vi "RetroParseGate.vi"(11 "Choose Directory":path) -> ()   [LabVIEW 2022 SP3]
panel:
  out "Raw data":i16[][](graph)
  out "Root Name":string
  out "File num":i32
  in  "Use Selected Files":bool
  in  "Listbox":i32[](listbox)
  in  "file ext":string="000"
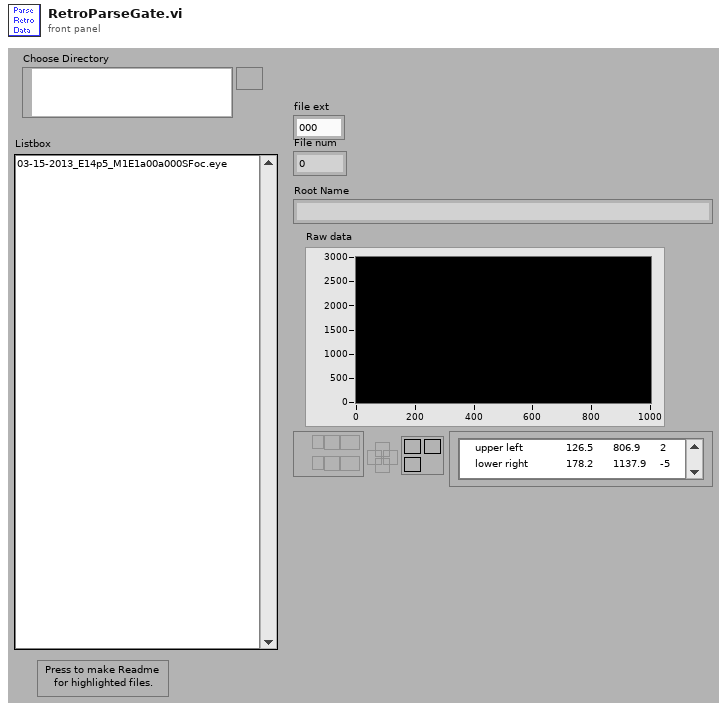
[diagram p1: front panel]
types:
  T1 = enum16{"open", "replace", "create", "open or create", "replace or create", "replace or create with confirmation"}
  T2 = enum16{"big-endian, network order", "native, host order", "little-endian"}
  T3 = cluster{"# rf points per line":u16, "# lines per scan":u16, "sample rate MHz":u16, "# A/D bits":i16, "# bytes per A/D":u16, "TGC Flag":u16, "A/D Type":string}
  T4 = typedef "Header.ctl" = cluster{"header info":cluster{"Header":string, "Head length":i16}, "A/D info":cluster{"# rf points per line":u16, "# lines per scan":u16, "sample rate MHz":u16, "# A/D bits":i16, "# bytes per A/D":u16, "TGC Flag":u16, "A/D Type":string}, "Tranducer Info":cluster{"bandwidth":sgl, "center freq":sgl, "start freq":sgl, "ID":i32}, "Scan Info":cluster{"delay":sgl, "pivot distance":sgl, "sector scan angle":sgl, "operator":string, "Scan Mode":string, "location":string}, "Time/Date Info":cluster{"date":string, "time":string}, "RF Info":cluster{"RF file name":string, "RF file att":string, "RF cal file name":string, "RF cal file att":string}, "Patient Info":cluster{"ID":string, "extended ID":string, "age":u16, "sex":string, "previously\nscanned":string, "PSA":sgl, "LOS":u8, "Ethnicty 2":u8, "Race":u8}, "Tissue Type":cluster{"organ":i16, "disease type":i16, "disease location":i16, "IQ_pts":u16, "RcvBuffer":u8, "RcvFrame":u16, "IQBuff":u8, "IQFrame":u16, "IQPage":u8}, "Votage scaling":cluster{"Digitizer (dB)":sgl, "Gain (dB)":sgl, "Atten (dB)":sgl}, "Comment":string, "Misc Info":cluster{"avg num":u16, "c speed":i16, "Div By or SF zones":i16, "XMIT CHS":u8, "RCV CHS":u8, "Xmit angle":sgl}, "Therapy Parameters":cluster{"Theraputic Freq (MHz)":sgl, "Time on (s)":sgl, "Therapy amplitude (mV)":sgl, "Lines Before":u16, "Lines After":u16}, "Scan Settings":cluster{"Energy (uJ or V)":u8, "Damp (Ohm) or Fc":u8, "HP Filt (KHz)":u8, "LP Filt (MHz)":u8, "Gain (db)":u8, "prf (kHz)":sgl, "Distance between\nscan lines (um)":u16, "Distance between\nscan planes (um)":u16, "Scan line gap (um)":sgl, "Scan plane gap (um)":sgl}, "Compression Parameters":cluster{"F1 (MHz)":sgl, "F2 (MHz)":sgl, "% taper":sgl, "duration":sgl}, "Patient Info Xtra":cluster{"First Name":string, "Last Name":string, "Notes":string}, "ROI Box":u16[]}
  T5 = cluster{"Energy (microJ)":u8, "Damping (In Ohm)":u8, "HP Filt(KHz) ":u8, "LP Filt (MHz)":u8, "Gain (db)":u8, "prf (kHz)":sgl, "Distance between\nscan lines (mm)":u16, "Distance between\nscan planes (mm)":u16}
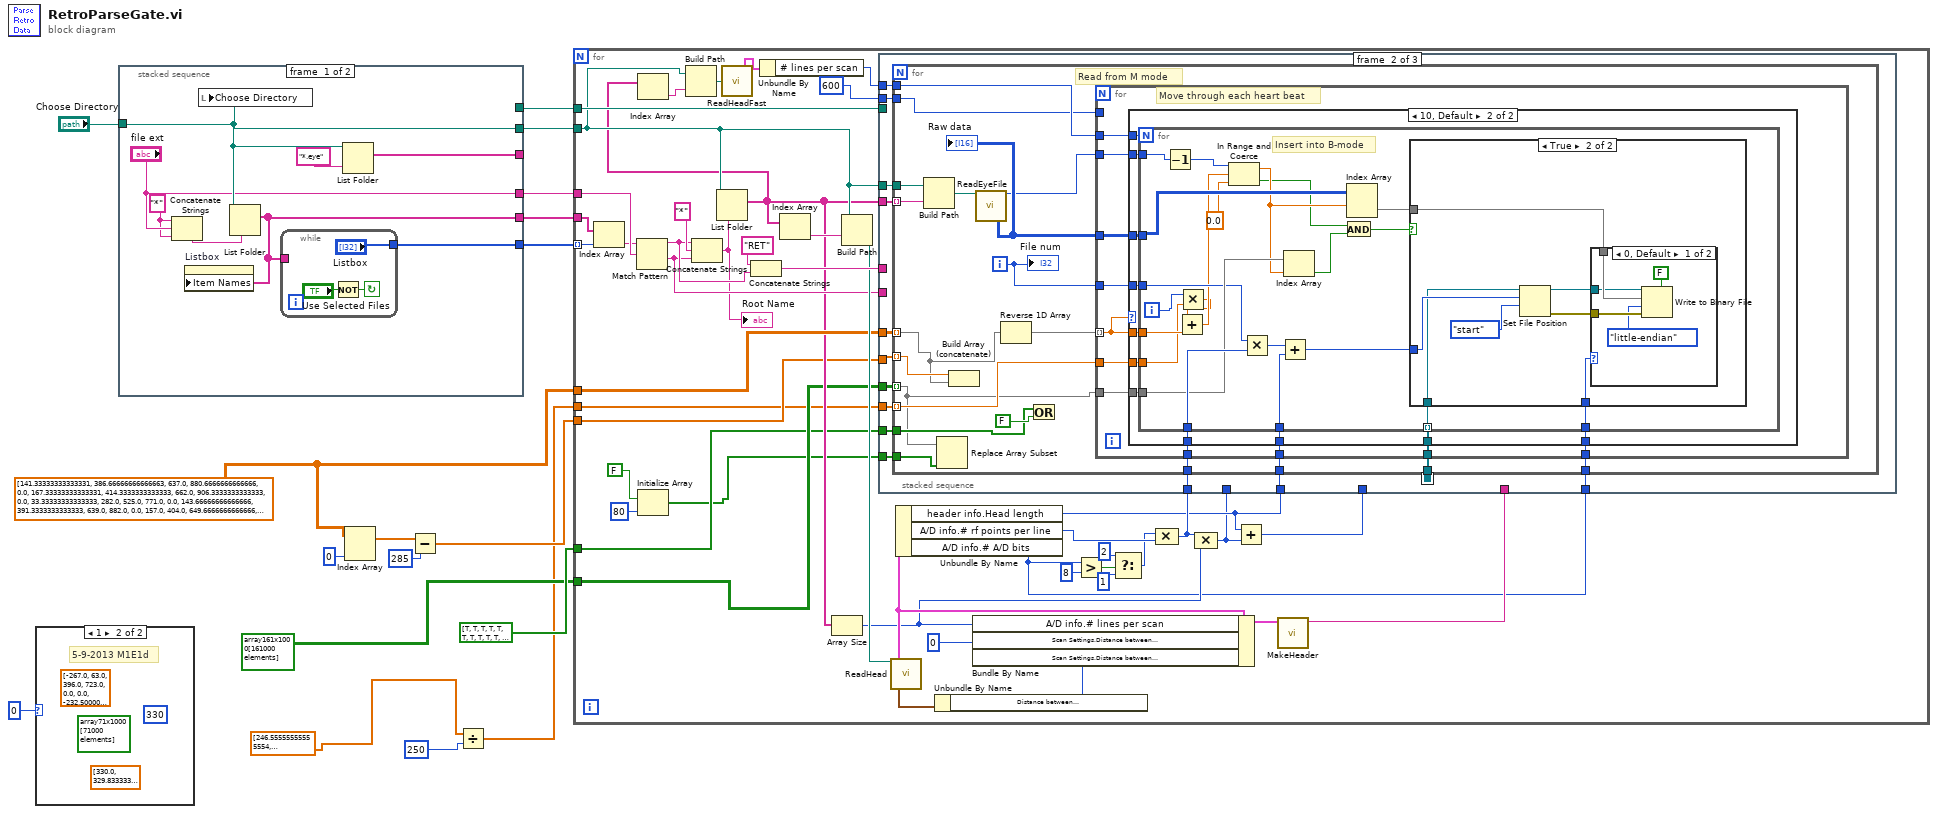
[diagram p0: block diagram]
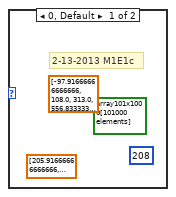
[diagram p2: hidden frame]
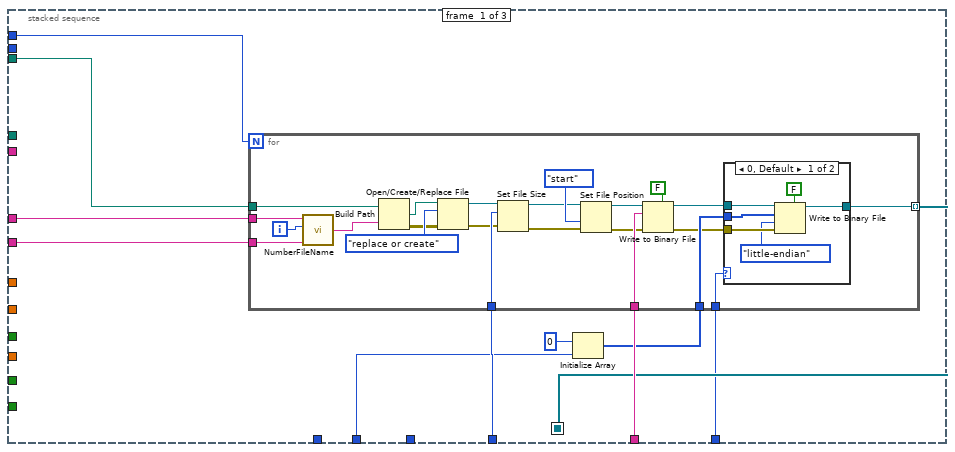
[diagram p3: hidden frame]
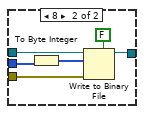
[diagram p4: hidden frame]
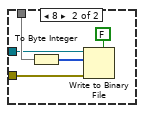
[diagram p7: hidden frame]
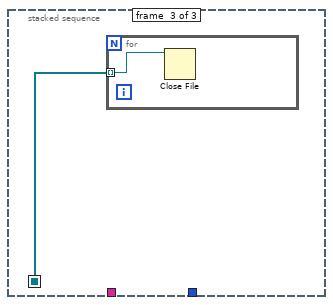
[diagram p8: hidden frame]
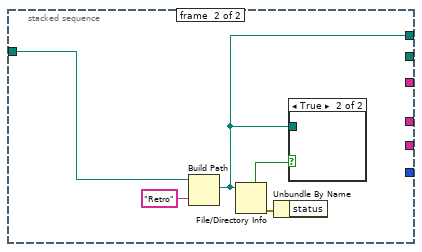
[diagram p9: hidden frame]
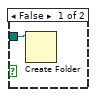
[diagram p10: hidden frame]
diagram:
  w3 = dbl[][] [[141.33333333333331, 386.66666666666663, 637.0, 880.6666666666666, 0.0], [167.33333333333331, 414.3333333333333, 662.0, 906.3333333333333, 0.0], [33.33333333333333, 282.0, 525.0, 771.0, 0.0], [143.66666666666666, 391.3333333333333, 639.0, 882.0, 0.0], [157.0, 404.0, 649.6666666666666, 893.6666666666666, 0.0], [157.66666666666666, 403.66666666666663, 651.0, 893.0, 0.0], [34.33333333333333, 283.66666666666663, 523.6666666666666, 767.6666666666666, 0.0], [120.0, 363.3333333333333, 607.6666666666666, 851.0, 0.0], [119.66666666666666, 364.0, 607.0, 853.0, 0.0], [117.0, 359.0, 604.3333333333333, 845.6666666666666, 0.0], [103.0, 347.3333333333333, 589.0, 833.6666666666666, 0.0], [124.0, 368.3333333333333, 612.6666666666666, 853.6666666666666, 0.0], [134.33333333333331, 376.0, 618.3333333333333, 860.6666666666666, 0.0], [120.0, 360.66666666666663, 604.3333333333333, 846.3333333333333, 0.0], [85.66666666666666, 328.66666666666663, 570.3333333333333, 816.3333333333333, 0.0], [96.66666666666666, 337.66666666666663, 579.6666666666666, 824.0, 0.0], [65.66666666666666, 306.66666666666663, 547.6666666666666, 789.6666666666666, 0.0], [26.333333333333332, 270.66666666666663, 512.3333333333333, 753.3333333333333, 0.0], [127.0, 369.0, 610.6666666666666, 854.6666666666666, 0.0], [142.33333333333331, 385.3333333333333, 627.0, 868.0, 0.0], [177.33333333333331, 420.0, 660.0, 901.6666666666666, 0.0], [192.33333333333331, 436.66666666666663, 678.3333333333333, 921.0, 0.0], [215.33333333333331, 458.3333333333333, 701.6666666666666, 944.3333333333333, 0.0], [20.333333333333332, 266.66666666666663, 508.66666666666663, 752.0, 0.0], [55.666666666666664, 300.3333333333333, 543.6666666666666, 787.3333333333333, 0.0], [73.33333333333333, 317.0, 560.0, 804.0, 0.0], [91.66666666666666, 336.3333333333333, 578.6666666666666, 820.6666666666666, 0.0], [120.33333333333333, 362.66666666666663, 606.0, 847.0, 0.0], [177.33333333333331, 419.0, 660.6666666666666, 902.0, 0.0], [191.66666666666666, 435.0, 673.3333333333333, 916.0, 0.0], [204.33333333333331, 445.0, 925.0, 0.0, 0.0], [235.0, 472.0, 712.0, 951.6666666666666, 0.0], [45.0, 282.66666666666663, 522.6666666666666, 760.3333333333333, 0.0], [66.66666666666666, 305.3333333333333, 547.0, 784.6666666666666, 0.0], [45.0, 282.0, 522.0, 763.3333333333333, 0.0], [77.0, 315.66666666666663, 556.0, 794.6666666666666, 0.0], [110.66666666666666, 349.3333333333333, 586.0, 827.0, 0.0], [135.33333333333331, 376.0, 612.3333333333333, 852.0, 0.0], [159.66666666666666, 400.3333333333333, 635.3333333333333, 877.6666666666666, 0.0], [141.0, 378.0, 615.6666666666666, 856.6666666666666, 0.0], [127.66666666666666, 366.0, 603.3333333333333, 843.3333333333333, 0.0], [149.66666666666666, 386.66666666666663, 622.6666666666666, 863.6666666666666, 0.0], [92.33333333333333, 328.0, 567.3333333333333, 808.3333333333333, 0.0], [79.66666666666666, 316.3333333333333, 553.6666666666666, 792.6666666666666, 0.0], [30.0, 266.3333333333333, 505.66666666666663, 742.0, 0.0], [9.333333333333332, 247.0, 486.66666666666663, 726.3333333333333, 960.0], [15.666666666666666, 252.33333333333331, 492.3333333333333, 727.6666666666666, 0.0], [197.0, 437.0, 672.0, 910.6666666666666, 0.0], [171.66666666666666, 411.3333333333333, 648.3333333333333, 887.3333333333333, 0.0], [149.0, 385.0, 623.3333333333333, 861.0, 0.0], [126.33333333333333, 363.3333333333333, 597.6666666666666, 837.0, 0.0], [111.0, 348.0, 581.6666666666666, 820.3333333333333, 0.0], [89.66666666666666, 321.66666666666663, 559.0, 799.0, 0.0], [77.33333333333333, 312.3333333333333, 548.6666666666666, 786.3333333333333, 0.0], [28.333333333333332, 262.3333333333333, 503.0, 737.0, 0.0], [92.66666666666666, 328.66666666666663, 567.0, 802.6666666666666, 0.0], [32.666666666666664, 267.0, 506.0, 740.3333333333333, 0.0], [188.0, 424.0, 658.3333333333333, 897.6666666666666, 0.0], [151.33333333333331, 386.66666666666663, 620.6666666666666, 860.6666666666666, 0.0], [341.3333333333333, 576.0, 0.0, 0.0, 0.0], [52.33333333333333, 285.3333333333333, 529.3333333333333, 759.6666666666666, 0.0], [238.33333333333331, 714.0, 949.0, 0.0, 0.0], [49.33333333333333, 285.0, 518.3333333333333, 757.6666666666666, 0.0], [80.33333333333333, 314.0, 552.0, 789.0, 0.0], [70.0, 305.0, 593.0, 777.0, 0.0], [228.66666666666666, 464.3333333333333, 701.3333333333333, 937.0, 0.0], [183.0, 654.3333333333333, 890.6666666666666, 0.0, 0.0], [134.66666666666666, 369.3333333333333, 603.0, 0.0, 0.0], [46.0, 282.0, 517.0, 752.0, 0.0], [231.66666666666666, 469.3333333333333, 702.0, 938.0, 0.0], [213.0, 679.6666666666666, 919.6666666666666, 0.0, 0.0], [27.666666666666664, 262.3333333333333, 498.0, 733.3333333333333, 966.3333333333333], [186.0, 421.66666666666663, 654.0, 892.6666666666666, 0.0], [143.0, 376.66666666666663, 611.3333333333333, 0.0, 0.0], [193.66666666666666, 662.3333333333333, 898.6666666666666, 0.0, 0.0], [120.0, 354.0, 589.0, 0.0, 0.0], [156.0, 623.0, 0.0, 0.0, 0.0], [314.66666666666663, 555.0, 0.0, 0.0, 0.0], [110.0, 344.0, 578.0, 815.0, 0.0], [134.0, 602.3333333333333, 0.0, 0.0, 0.0], [170.33333333333331, 638.0, 0.0, 0.0, 0.0], [131.33333333333331, 366.0, 600.6666666666666, 833.3333333333333, 0.0], [5.333333333333333, 237.33333333333331, 472.66666666666663, 709.3333333333333, 939.3333333333333], [164.66666666666666, 401.66666666666663, 634.6666666666666, 866.0, 0.0], [165.66666666666666, 399.0, 633.0, 866.0, 0.0], [150.33333333333331, 384.0, 620.3333333333333, 853.6666666666666, 0.0], [102.33333333333333, 336.0, 570.6666666666666, 804.6666666666666, 0.0], [65.66666666666666, 300.0, 532.6666666666666, 767.3333333333333, 0.0], [52.0, 288.3333333333333, 519.6666666666666, 752.6666666666666, 0.0], [56.0, 293.3333333333333, 525.0, 756.6666666666666, 0.0], [225.33333333333331, 458.3333333333333, 703.3333333333333, 926.0, 0.0], [170.33333333333331, 402.66666666666663, 636.6666666666666, 873.3333333333333, 0.0], [115.66666666666666, 347.3333333333333, 582.6666666666666, 815.6666666666666, 0.0], [27.666666666666664, 261.66666666666663, 496.0, 729.3333333333333, 962.3333333333333], [188.66666666666666, 420.3333333333333, 655.3333333333333, 889.0, 0.0], [152.0, 385.66666666666663, 618.3333333333333, 853.6666666666666, 0.0], [159.66666666666666, 391.0, 626.0, 858.6666666666666, 0.0], [158.0, 392.66666666666663, 624.3333333333333, 858.3333333333333, 0.0], [103.33333333333333, 336.66666666666663, 570.6666666666666, 803.0, 0.0], [39.666666666666664, 275.66666666666663, 506.66666666666663, 751.6666666666666, 0.0], [194.0, 426.3333333333333, 659.6666666666666, 893.6666666666666, 0.0], [139.33333333333331, 371.3333333333333, 604.0, 837.3333333333333, 0.0], [85.66666666666666, 319.3333333333333, 553.3333333333333, 784.6666666666666, 0.0], [220.0, 453.0, 687.3333333333333, 920.6666666666666, 0.0], [118.66666666666666, 352.66666666666663, 586.6666666666666, 819.3333333333333, 0.0], [40.0, 274.66666666666663, 506.66666666666663, 738.3333333333333, 0.0], [16.333333333333332, 249.0, 485.0, 716.3333333333333, 950.3333333333333], [200.33333333333331, 434.0, 668.0, 900.3333333333333, 0.0], [102.0, 333.66666666666663, 566.0, 797.6666666666666, 0.0], [32.33333333333333, 267.3333333333333, 499.0, 734.6666666666666, 964.0], [208.33333333333331, 443.3333333333333, 675.3333333333333, 908.3333333333333, 0.0], [94.0, 326.3333333333333, 560.3333333333333, 794.6666666666666, 0.0], [205.0, 438.0, 671.3333333333333, 904.6666666666666, 0.0], [90.66666666666666, 328.3333333333333, 557.6666666666666, 790.6666666666666, 0.0], [206.66666666666666, 439.3333333333333, 672.6666666666666, 907.3333333333333, 0.0], [149.0, 383.3333333333333, 613.0, 849.6666666666666, 0.0], [74.66666666666666, 303.66666666666663, 540.0, 775.6666666666666, 0.0], [193.33333333333331, 427.3333333333333, 659.3333333333333, 893.3333333333333, 0.0], [75.33333333333333, 307.66666666666663, 541.3333333333333, 772.6666666666666, 0.0], [227.66666666666666, 459.3333333333333, 927.0, 0.0, 0.0], [171.0, 404.66666666666663, 637.0, 869.6666666666666, 0.0], [67.0, 533.3333333333333, 766.3333333333333, 0.0, 0.0], [145.33333333333331, 376.66666666666663, 611.3333333333333, 846.3333333333333, 0.0], [220.0, 452.0, 685.0, 917.3333333333333, 0.0], [140.66666666666666, 373.0, 605.6666666666666, 839.6666666666666, 0.0], [47.33333333333333, 291.0, 515.3333333333333, 750.3333333333333, 0.0], [184.33333333333331, 419.0, 651.3333333333333, 886.0, 0.0], [102.0, 335.0, 567.0, 800.6666666666666, 0.0], [166.0, 399.3333333333333, 630.3333333333333, 864.0, 0.0], [10.0, 243.33333333333331, 476.66666666666663, 709.0, 943.6666666666666], [103.33333333333333, 335.66666666666663, 570.3333333333333, 802.6666666666666, 0.0], [12.0, 245.0, 477.3333333333333, 711.6666666666666, 946.0], [79.0, 318.66666666666663, 547.3333333333333, 780.0, 0.0], [158.33333333333331, 392.0, 626.3333333333333, 859.6666666666666, 0.0], [21.0, 254.33333333333331, 490.0, 721.6666666666666, 954.6666666666666], [139.33333333333331, 369.66666666666663, 604.0, 836.6666666666666, 0.0], [223.33333333333331, 458.3333333333333, 691.6666666666666, 924.3333333333333, 0.0], [38.0, 272.66666666666663, 504.3333333333333, 741.6666666666666, 0.0], [54.33333333333333, 522.0, 759.6666666666666, 0.0, 0.0], [144.33333333333331, 376.3333333333333, 611.3333333333333, 846.6666666666666, 0.0], [12.0, 244.33333333333331, 478.66666666666663, 711.3333333333333, 945.6666666666666], [78.0, 544.0, 778.3333333333333, 0.0, 0.0], [131.33333333333331, 363.3333333333333, 597.0, 830.0, 0.0], [141.0, 373.0, 606.6666666666666, 842.0, 0.0], [188.33333333333331, 422.3333333333333, 654.3333333333333, 887.3333333333333, 0.0], [53.666666666666664, 521.0, 758.0, 0.0, 0.0], [134.33333333333331, 365.3333333333333, 600.0, 832.6666666666666, 0.0], [218.33333333333331, 451.66666666666663, 686.6666666666666, 920.0, 0.0], [8.666666666666666, 240.0, 473.3333333333333, 708.3333333333333, 940.3333333333333], [217.66666666666666, 451.66666666666663, 686.6666666666666, 917.3333333333333, 0.0], [238.66666666666666, 470.0, 705.6666666666666, 940.0, 0.0], [50.33333333333333, 287.3333333333333, 519.3333333333333, 762.6666666666666, 0.0], [109.0, 343.66666666666663, 574.6666666666666, 810.0, 0.0], [160.0, 392.66666666666663, 626.6666666666666, 859.3333333333333, 0.0], [170.66666666666666, 403.3333333333333, 639.0, 869.0, 0.0], [139.33333333333331, 371.0, 836.0, 0.0, 0.0], [152.33333333333331, 383.3333333333333, 621.6666666666666, 851.6666666666666, 0.0], [236.33333333333331, 471.66666666666663, 700.6666666666666, 935.6666666666666, 0.0], [23.666666666666664, 258.0, 491.66666666666663, 725.6666666666666, 957.0], [226.33333333333331, 459.66666666666663, 693.3333333333333, 924.6666666666666, 0.0], [212.33333333333331, 443.0, 677.0, 911.0, 0.0]] ("Beat INput")
  n1 = case shown="1" 0 {
    frame 0, Default {
      (unwired) 208
      (unwired) dbl[] [205.91666666666666, 210.27777777777777, 205.88888888888889, 208.66666666666666, 207.25, 211.72222222222223, 206.77777777777774, 211.54166666666666, 208.83333333333331, 212.27777777777774, 215.55555555555554, 212.25, 215.7222222222222, 217.04166666666666, 213.38888888888889, 217.875, 218.16666666666666, 163.375, 220.87499999999997, 219.77777777777777, 221.94444444444446, 221.5, 221.5, 224.27777777777777, 224.27777777777777, 224.5, 224.94444444444443, 222.54166666666666, 223.27777777777774, 223.625, 227.88888888888886, 223.88888888888886, 222.77777777777777, 222.83333333333331, 222.20833333333331, 223.16666666666666, 222.91666666666666, 223.11111111111111, 221.91666666666669, 223.33333333333331, 221.05555555555554, 221.7222222222222, 220.16666666666666, 221.70833333333331, 222.72222222222223, 220.77777777777774, 222.11111111111111, 220.66666666666666, 223.04166666666666, 223.27777777777777, 223.2222222222222, 223.66666666666666, 222.61111111111111, 227.27777777777774, 223.95833333333331, 225.88888888888886, 223.875, 226.45833333333334, 227.7222222222222, 224.88888888888889, 224.83333333333334, 223.375, 224.75, 223.0, 223.94444444444446, 223.54166666666666, 223.61111111111111, 225.94444444444443, 226.0, 225.87499999999997, 228.66666666666666, 230.72222222222223, 230.33333333333334, 226.20833333333334, 232.0, 231.55555555555554, 230.70833333333334, 232.66666666666666, 231.94444444444443, 230.2222222222222, 228.83333333333331, 229.79166666666666, 234.27777777777777, 233.16666666666666, 232.77777777777774, 229.16666666666666, 228.6111111111111, 234.55555555555557, 232.20833333333331, 232.05555555555557, 229.61111111111111, 231.6111111111111, 230.29166666666666, 230.29166666666669, 228.61111111111111, 231.1111111111111, 231.91666666666666, 232.49999999999997, 232.27777777777777, 231.27777777777774, 230.55555555555557] ("Array")
      (unwired) bool[][] array101x1000[101000 elements] ("Resp Gate")
      (unwired) dbl[][] [[-97.91666666666666, 108.0, 313.0, 556.8333333333333, 720.3333333333333, 931.6666666666666, 0.0], [-29.611111111111114, 180.66666666666666, 392.3333333333333, 603.5, 811.5, 0.0, 0.0], [-44.888888888888886, 161.0, 365.8333333333333, 624.1666666666666, 778.6666666666666, 0.0, 0.0], [-50.0, 158.66666666666666, 368.8333333333333, 573.1666666666666, 784.6666666666666, 0.0, 0.0], [-131.91666666666669, 75.33333333333333, 285.16666666666663, 492.66666666666663, 699.5, 904.3333333333333, 0.0], [-40.388888888888914, 171.33333333333331, 383.3333333333333, 596.0, 806.5, 0.0, 0.0], [-14.777777777777743, 192.0, 403.3333333333333, 636.8333333333333, 812.3333333333333, 0.0, 0.0], [-102.04166666666666, 109.5, 323.66666666666663, 545.1666666666666, 745.8333333333333, 955.6666666666666, 0.0], [-136.5, 72.33333333333333, 283.0, 493.0, 695.1666666666666, 907.6666666666666, 0.0], [-1.277777777777743, 211.0, 423.66666666666663, 635.1666666666666, 847.8333333333333, 0.0, 0.0], [3.444444444444457, 219.0, 434.3333333333333, 650.3333333333333, 865.6666666666666, 0.0, 0.0], [-89.41666666666667, 122.83333333333333, 330.3333333333333, 543.0, 758.6666666666666, 971.8333333333333, 0.0], [-73.2222222222222, 142.5, 358.5, 576.1666666666666, 789.6666666666666, 0.0, 0.0], [-196.70833333333331, 20.333333333333332, 238.16666666666666, 452.66666666666663, 671.3333333333333, 888.5, 0.0], [-9.888888888888886, 203.5, 440.8333333333333, 628.0, 843.6666666666666, 0.0, 0.0], [-117.875, 100.0, 318.5, 535.1666666666666, 752.0, 971.5, 0.0], [-141.66666666666666, 76.5, 316.3333333333333, 512.1666666666666, 730.3333333333333, 949.1666666666666, 0.0], [-37.54166666666667, 125.83333333333333, 345.0, 387.8333333333333, 559.1666666666666, 779.3333333333333, 0.0], [-197.54166666666663, 23.333333333333332, 245.66666666666666, 491.0, 686.3333333333333, 906.8333333333333, 0.0], [-24.444444444444457, 195.33333333333331, 416.0, 633.6666666666666, 854.6666666666666, 0.0, 0.0], [-185.2777777777778, 36.666666666666664, 258.66666666666663, 480.66666666666663, 702.5, 0.0, 0.0], [4.666666666666657, 226.16666666666666, 446.16666666666663, 669.6666666666666, 890.6666666666666, 0.0, 0.0], [-114.83333333333334, 106.66666666666666, 328.0, 547.6666666666666, 771.1666666666666, 0.0, 0.0], [-30.111111111111114, 194.16666666666666, 455.8333333333333, 643.3333333333333, 867.0, 0.0, 0.0], [-79.61111111111111, 144.66666666666666, 371.5, 595.8333333333333, 817.5, 0.0, 0.0], [-150.16666666666669, 74.33333333333333, 299.3333333333333, 524.3333333333333, 747.0, 972.3333333333333, 0.0], [-125.1111111111111, 99.83333333333333, 323.66666666666663, 547.8333333333333, 774.6666666666666, 0.0, 0.0], [-160.875, 61.666666666666664, 283.3333333333333, 507.5, 730.0, 951.8333333333333, 0.0], [-59.77777777777774, 163.5, 387.8333333333333, 610.3333333333333, 833.3333333333333, 0.0, 0.0], [-151.625, 72.0, 296.0, 549.0, 743.8333333333333, 966.5, 0.0], [-70.7222222222222, 157.16666666666666, 380.3333333333333, 603.8333333333333, 840.8333333333333, 0.0, 0.0], [-67.7222222222222, 156.16666666666666, 378.8333333333333, 616.6666666666666, 827.8333333333333, 0.0, 0.0], [-88.94444444444446, 133.83333333333331, 359.3333333333333, 585.5, 802.1666666666666, 0.0, 0.0], [-128.16666666666666, 94.66666666666666, 316.3333333333333, 539.5, 763.1666666666666, 0.0, 0.0], [-168.875, 53.33333333333333, 276.0, 519.1666666666666, 719.3333333333333, 942.1666666666666, 0.0], [-87.33333333333334, 135.83333333333331, 361.16666666666663, 581.8333333333333, 805.3333333333333, 0.0, 0.0], [-205.91666666666666, 17.0, 239.33333333333331, 465.0, 686.8333333333333, 908.6666666666666, 0.0], [-74.44444444444446, 148.66666666666666, 372.3333333333333, 598.8333333333333, 818.0, 0.0, 0.0], [-134.08333333333337, 87.83333333333333, 308.3333333333333, 530.5, 752.6666666666666, 975.5, 0.0], [-85.66666666666666, 137.66666666666666, 360.3333333333333, 583.6666666666666, 807.6666666666666, 0.0, 0.0], [-100.88888888888889, 120.16666666666666, 342.16666666666663, 563.1666666666666, 783.3333333333333, 0.0, 0.0], [-59.2222222222222, 162.5, 386.3333333333333, 607.3333333333333, 827.6666666666666, 0.0, 0.0], [-23.166666666666657, 197.0, 415.16666666666663, 636.0, 857.5, 0.0, 0.0], [-204.70833333333331, 17.0, 237.16666666666666, 498.8333333333333, 682.8333333333333, 903.8333333333333, 0.0], [-18.388888888888914, 204.33333333333331, 426.5, 649.0, 872.5, 0.0, 0.0], [-83.77777777777774, 137.0, 359.66666666666663, 576.1666666666666, 799.3333333333333, 0.0, 0.0], [-36.94444444444446, 185.16666666666666, 406.3333333333333, 629.3333333333333, 851.5, 0.0, 0.0], [-99.33333333333333, 121.33333333333333, 342.3333333333333, 562.0, 783.3333333333333, 0.0, 0.0], [-166.04166666666666, 57.0, 279.8333333333333, 517.3333333333333, 724.6666666666666, 949.1666666666666, 0.0], [-12.444444444444457, 210.83333333333331, 431.0, 654.3333333333333, 880.6666666666666, 0.0, 0.0], [-43.55555555555554, 179.66666666666666, 400.66666666666663, 627.1666666666666, 849.3333333333333, 0.0, 0.0], [-100.16666666666666, 123.5, 347.0, 573.6666666666666, 794.5, 0.0, 0.0], [-125.27777777777779, 97.33333333333333, 319.0, 543.3333333333333, 765.1666666666666, 0.0, 0.0], [-103.27777777777774, 124.0, 352.3333333333333, 579.5, 805.8333333333333, 0.0, 0.0], [-208.45833333333331, 15.5, 239.66666666666666, 480.16666666666663, 684.6666666666666, 911.3333333333333, 0.0], [-53.2222222222222, 172.66666666666666, 398.66666666666663, 623.0, 850.3333333333333, 0.0, 0.0], [-187.70833333333334, 36.166666666666664, 261.0, 485.3333333333333, 709.1666666666666, 931.6666666666666, 0.0], [-159.29166666666669, 67.16666666666666, 293.16666666666663, 527.8333333333333, 747.6666666666666, 973.0, 0.0], [-36.05555555555554, 191.66666666666666, 420.5, 645.8333333333333, 874.8333333333333, 0.0, 0.0], [-43.388888888888886, 181.5, 408.0, 631.3333333333333, 856.1666666666666, 0.0, 0.0], [2.166666666666657, 227.0, 467.8333333333333, 678.8333333333333, 901.5, 0.0, 0.0], [-145.20833333333334, 78.16666666666666, 301.66666666666663, 547.6666666666666, 747.1666666666666, 971.6666666666666, 0.0], [-182.08333333333334, 42.666666666666664, 272.3333333333333, 497.5, 720.0, 941.6666666666666, 0.0], [-47.33333333333334, 175.66666666666666, 398.8333333333333, 623.5, 844.6666666666666, 0.0, 0.0], [-41.7777777777778, 182.16666666666666, 404.8333333333333, 626.6666666666666, 854.0, 0.0, 0.0], [-198.04166666666666, 25.5, 247.83333333333331, 471.16666666666663, 696.8333333333333, 919.6666666666666, 0.0], [-29.444444444444457, 194.16666666666666, 419.16666666666663, 641.0, 865.0, 0.0, 0.0], [-7.611111111111114, 218.33333333333331, 444.3333333333333, 669.0, 896.1666666666666, 0.0, 0.0], [-95.5, 130.5, 353.8333333333333, 583.0, 808.5, 0.0, 0.0], [-203.04166666666663, 22.833333333333332, 250.66666666666666, 471.66666666666663, 699.1666666666666, 926.3333333333333, 0.0], [-199.0, 29.666666666666664, 262.3333333333333, 502.8333333333333, 716.5, 944.3333333333333, 0.0], [-29.888888888888914, 200.83333333333331, 430.3333333333333, 661.6666666666666, 893.0, 0.0, 0.0], [-85.33333333333334, 145.0, 377.16666666666663, 604.0, 836.0, 0.0, 0.0], [-192.54166666666669, 33.666666666666664, 245.16666666666666, 475.8333333333333, 708.6666666666666, 938.5, 0.0], [-188.16666666666669, 43.83333333333333, 278.16666666666663, 516.8333333333333, 741.1666666666666, 971.8333333333333, 0.0], [-75.55555555555554, 156.0, 387.0, 617.6666666666666, 850.6666666666666, 0.0, 0.0], [-190.54166666666669, 40.166666666666664, 269.5, 504.3333333333333, 734.5, 963.0, 0.0], [-36.33333333333334, 196.33333333333331, 426.66666666666663, 659.0, 894.3333333333333, 0.0, 0.0], [-101.94444444444443, 130.0, 362.16666666666663, 592.6666666666666, 825.8333333333333, 0.0, 0.0], [-165.05555555555554, 65.16666666666666, 293.3333333333333, 521.6666666666666, 755.8333333333333, 0.0, 0.0], [-8.166666666666657, 220.66666666666666, 458.3333333333333, 677.5, 907.1666666666666, 0.0, 0.0], [-216.125, 13.666666666666666, 243.0, 470.3333333333333, 702.0, 932.8333333333333, 0.0], [-85.11111111111111, 149.16666666666666, 382.0, 616.0, 852.0, 0.0, 0.0], [-116.83333333333333, 116.33333333333333, 353.3333333333333, 585.5, 815.8333333333333, 0.0, 0.0], [-1.277777777777743, 231.5, 462.5, 696.0, 929.8333333333333, 0.0, 0.0], [-122.66666666666666, 106.5, 336.8333333333333, 560.1666666666666, 794.0, 0.0, 0.0], [-148.77777777777777, 79.83333333333333, 306.16666666666663, 544.8333333333333, 765.6666666666666, 0.0, 0.0], [-122.72222222222224, 111.83333333333333, 342.16666666666663, 581.6666666666666, 815.5, 0.0, 0.0], [-197.70833333333331, 34.5, 269.16666666666663, 515.5, 732.0, 963.3333333333333, 0.0], [-29.722222222222257, 202.33333333333331, 430.3333333333333, 665.8333333333333, 898.5, 0.0, 0.0], [-45.2777777777778, 184.33333333333331, 412.16666666666663, 653.1666666666666, 873.1666666666666, 0.0, 0.0], [-89.11111111111109, 142.5, 375.5, 606.8333333333333, 837.3333333333333, 0.0, 0.0], [-215.125, 15.166666666666666, 246.0, 473.66666666666663, 703.0, 936.3333333333333, 0.0], [-184.45833333333337, 45.83333333333333, 275.66666666666663, 506.5, 738.0, 967.0, 0.0], [-91.7777777777778, 136.83333333333331, 365.8333333333333, 592.6666666666666, 822.6666666666666, 0.0, 0.0], [-111.11111111111109, 120.0, 353.0, 583.0, 813.3333333333333, 0.0, 0.0], [-205.41666666666666, 26.5, 257.5, 496.3333333333333, 723.8333333333333, 954.1666666666666, 0.0], [-78.16666666666666, 154.33333333333331, 386.16666666666663, 618.8333333333333, 851.8333333333333, 0.0, 0.0], [-16.611111111111114, 215.66666666666666, 440.8333333333333, 677.8333333333333, 912.5, 0.0, 0.0], [-50.27777777777774, 181.0, 413.5, 641.1666666666666, 874.8333333333333, 0.0, 0.0], [-19.222222222222257, 211.33333333333331, 440.8333333333333, 675.1666666666666, 903.0, 0.0, 0.0]] ("Beat Ref Marks")
      # "2-13-2013 M1E1c"
    }
    frame 1 {
      (unwired) 330
      (unwired) bool[][] array71x1000[71000 elements] ("Resp Gate")
      (unwired) dbl[] [330.0, 329.83333333333337, 327.66666666666663, 333.3333333333333, 333.1666666666667, 335.3333333333333, 332.16666666666663, 331.5, 331.0, 330.33333333333326, 332.83333333333337, 335.3333333333333, 333.33333333333326, 336.33333333333337, 335.0, 334.6666666666667, 337.33333333333337, 341.16666666666663, 338.99999999999994, 338.6666666666667, 338.83333333333337, 339.5, 334.66666666666663, 339.16666666666663, 338.0, 335.5, 338.5, 336.6666666666667, 339.5, 337.33333333333337, 332.3333333333333, 334.6666666666667, 332.0, 331.0, 332.0, 332.0, 333.66666666666663, 332.8333333333333, 334.6666666666667, 333.33333333333337, 333.33333333333337, 330.16666666666663, 330.66666666666663, 329.83333333333337, 329.16666666666663, 330.16666666666663, 329.3333333333333, 333.66666666666663, 330.8333333333333, 330.33333333333337, 328.83333333333337, 329.83333333333337, 332.66666666666663, 331.6666666666667, 327.33333333333337, 329.33333333333337, 333.16666666666663, 331.6666666666667, 334.16666666666663, 332.33333333333337, 331.33333333333337, 334.0, 333.33333333333337, 334.83333333333326, 337.6666666666667, 334.83333333333337, 332.33333333333337, 334.66666666666663, 334.3333333333333, 332.0, 334.66666666666663] ("Array")
      (unwired) dbl[][] [[-267.0, 63.0, 396.0, 723.0, 0.0, 0.0], [-232.50000000000006, 97.33333333333333, 428.0, 757.0, 0.0, 0.0], [-226.33333333333331, 101.33333333333333, 427.66666666666663, 756.6666666666666, 0.0, 0.0], [-153.66666666666666, 179.66666666666666, 516.3333333333333, 846.3333333333333, 0.0, 0.0], [-173.50000000000003, 159.66666666666666, 493.0, 826.0, 0.0, 0.0], [-109.33333333333331, 226.0, 560.0, 896.6666666666666, 0.0, 0.0], [-71.83333333333331, 260.3333333333333, 591.3333333333333, 924.6666666666666, 0.0, 0.0], [-324.1666666666667, 7.333333333333333, 339.66666666666663, 670.3333333333333, 0.0, 0.0], [-280.6666666666667, 50.33333333333333, 383.3333333333333, 712.3333333333333, 0.0, 0.0], [7.6666666666667425, 338.0, 668.3333333333333, 0.0, 0.0, 0.0], [-124.50000000000006, 208.33333333333331, 542.3333333333333, 874.0, 0.0, 0.0], [-282.3333333333333, 53.0, 388.66666666666663, 723.6666666666666, 0.0, 0.0], [-165.6666666666666, 167.66666666666666, 500.3333333333333, 834.3333333333333, 0.0, 0.0], [-2.6666666666667425, 333.66666666666663, 670.0, 0.0, 0.0, 0.0], [-198.66666666666669, 136.33333333333331, 471.0, 806.3333333333333, 0.0, 0.0], [-65.00000000000006, 269.66666666666663, 603.0, 939.0, 0.0, 0.0], [-180.00000000000006, 157.33333333333331, 494.0, 832.0, 0.0, 0.0], [-311.16666666666663, 30.0, 370.0, 712.3333333333333, 0.0, 0.0], [-37.66666666666663, 301.3333333333333, 640.3333333333333, 0.0, 0.0, 0.0], [-68.00000000000006, 270.66666666666663, 610.6666666666666, 948.0, 0.0, 0.0], [-238.50000000000006, 100.33333333333333, 440.3333333333333, 778.0, 0.0, 0.0], [-244.16666666666669, 95.33333333333333, 436.3333333333333, 774.3333333333333, 0.0, 0.0], [-324.99999999999994, 9.666666666666666, 344.0, 679.0, 0.0, 0.0], [-150.83333333333331, 188.33333333333331, 529.0, 866.6666666666666, 0.0, 0.0], [-159.0, 179.0, 520.0, 855.0, 0.0, 0.0], [-301.1666666666667, 34.33333333333333, 366.66666666666663, 705.3333333333333, 0.0, 0.0], [-160.16666666666669, 178.33333333333331, 519.0, 855.3333333333333, 0.0, 0.0], [-219.00000000000003, 117.66666666666666, 451.66666666666663, 791.0, 0.0, 0.0], [-152.16666666666669, 187.33333333333331, 524.3333333333333, 866.3333333333333, 0.0, 0.0], [-221.00000000000006, 116.33333333333333, 450.3333333333333, 791.0, 0.0, 0.0], [9.0, 341.3333333333333, 673.6666666666666, 0.0, 0.0, 0.0], [-55.00000000000006, 279.66666666666663, 615.3333333333333, 949.0, 0.0, 0.0], [-292.0, 40.0, 374.3333333333333, 704.0, 0.0, 0.0], [-262.0, 69.0, 399.0, 731.0, 0.0, 0.0], [-48.33333333333337, 283.66666666666663, 616.0, 947.6666666666666, 0.0, 0.0], [-92.66666666666669, 239.33333333333331, 575.6666666666666, 903.3333333333333, 0.0, 0.0], [-173.99999999999997, 159.66666666666666, 487.3333333333333, 827.0, 0.0, 0.0], [-58.833333333333314, 274.0, 608.6666666666666, 939.6666666666666, 0.0, 0.0], [-19.33333333333337, 315.3333333333333, 650.0, 0.0, 0.0, 0.0], [-105.00000000000006, 228.33333333333331, 564.3333333333333, 895.0, 0.0, 0.0], [-92.00000000000006, 241.33333333333331, 574.0, 908.0, 0.0, 0.0], [-260.16666666666663, 70.0, 397.66666666666663, 730.3333333333333, 0.0, 0.0], [-86.33333333333331, 244.33333333333331, 577.3333333333333, 905.6666666666666, 0.0, 0.0], [-100.50000000000006, 229.33333333333331, 561.3333333333333, 889.0, 0.0, 0.0], [-222.16666666666663, 107.0, 439.3333333333333, 765.3333333333333, 0.0, 0.0], [-42.833333333333314, 287.3333333333333, 617.3333333333333, 947.6666666666666, 0.0, 0.0], [-56.666666666666686, 272.66666666666663, 608.0, 931.3333333333333, 0.0, 0.0], [-298.99999999999994, 34.666666666666664, 368.66666666666663, 702.0, 0.0, 0.0], [-265.8333333333333, 65.0, 398.3333333333333, 726.6666666666666, 0.0, 0.0], [-45.00000000000006, 285.3333333333333, 618.0, 946.0, 0.0, 0.0], [-108.50000000000006, 220.33333333333331, 552.3333333333333, 878.0, 0.0, 0.0], [-128.50000000000006, 201.33333333333331, 530.6666666666666, 861.0, 0.0, 0.0], [-173.66666666666663, 159.0, 488.66666666666663, 824.3333333333333, 0.0, 0.0], [-198.00000000000003, 133.66666666666666, 461.66666666666663, 797.0, 0.0, 0.0], [-13.666666666666742, 313.66666666666663, 641.0, 0.0, 0.0, 0.0], [8.333333333333258, 337.66666666666663, 667.0, 0.0, 0.0, 0.0], [-296.49999999999994, 36.666666666666664, 368.3333333333333, 703.0, 0.0, 0.0], [-255.00000000000003, 76.66666666666666, 406.0, 740.0, 0.0, 0.0], [-288.8333333333333, 45.33333333333333, 381.3333333333333, 713.6666666666666, 0.0, 0.0], [-91.00000000000006, 241.33333333333331, 573.3333333333333, 906.0, 0.0, 0.0], [-169.00000000000006, 162.33333333333331, 492.66666666666663, 825.0, 0.0, 0.0], [-321.3333333333333, 12.666666666666666, 346.66666666666663, 680.6666666666666, 0.0, 0.0], [-265.00000000000006, 68.33333333333333, 400.0, 735.0, 0.0, 0.0], [-198.1666666666666, 136.66666666666666, 472.3333333333333, 806.3333333333333, 0.0, 0.0], [-201.00000000000003, 136.66666666666666, 470.66666666666663, 812.0, 0.0, 0.0], [-230.50000000000006, 104.33333333333333, 436.0, 774.0, 0.0, 0.0], [-20.666666666666742, 311.66666666666663, 644.0, 0.0, 0.0, 0.0], [-168.33333333333331, 166.33333333333331, 503.0, 835.6666666666666, 0.0, 0.0], [-300.3333333333333, 34.0, 369.0, 702.6666666666666, 0.0, 0.0], [-67.33333333333337, 264.66666666666663, 593.3333333333333, 928.6666666666666, 0.0, 0.0], [-296.99999999999994, 37.666666666666664, 366.3333333333333, 707.0, 0.0, 0.0]] ("Beat Ref Marks")
      # "5-9-2013 M1E1d"
    }
  }
  n2 = stacked-sequence {
    tunnel: "Choose Directory" -> [w21 w33]
    tunnel: [w24 _] -> _
    tunnel: [w23 _] -> w16
    tunnel: [w22 _] -> w15
    tunnel: ["file ext" _] -> w14
    tunnel: [w21 _] -> w13
    tunnel: [_ w29] -> w12
    frame #0 {
      w18 = "*" ("prompt")
      n3 = Concatenate Strings(w18, "file ext", w18) -> (w19:string)
      n4 = local write "Choose Directory"(w21) -> ()
      n5 = List Folder(path=w21, pattern=w19) -> (filenames=w22:string[])  [unwired: 1 in, 4 out]
      n6 = property on="Listbox" class="LstBox (strict)"("Item Names"=w22) -> ()  [unwired: 2 in, 2 out]
      n7 = while {
        tunnel: ["Listbox"] -> w23
        tunnel: w22 -> [_]
        stop <- w28 continue-if-true
        n8 = Not(x="Use Selected Files") -> (.not. x?=w28:bool)
      }
      n9 = List Folder(path=w21, pattern="*.eye" ("prompt")) -> (filenames=w24:string[])  [unwired: 1 in, 4 out]
    }
    frame #1 {
      n10 = Build Path(base path=w33, name or relative path="Retro") -> (appended path=w29:path)
      n11 = File/Directory Info(path=w29) -> (directory=w31:bool, error out=w30:errorcluster)  [unwired: 1 in, 5 out]
      n12 = Unbundle By Name(w30) -> ()  [unwired: 1 out]
      n13 = case shown="True" w31 {
        tunnel: w29 -> [w34 _]
        frame False {
          n14 = Create Folder(path (use dialog)=w34) -> ()  [unwired: 1 in, 4 out]
        }
        frame True {
        }
      }
    }
  }
  n15 = Index Array(array=w3, index (col)=0 ("disabled index (col)")) -> (element=w9:dbl[])  [unwired: 1 in]
  n16 = Subtract(x=w9, y=285) -> (x-y=w8:dbl[])
  n17 = Divide(x=dbl[] [246.55555555555554, 246.44444444444443, 245.88888888888889, 245.55555555555557, 245.88888888888889, 244.55555555555557, 244.44444444444443, 243.66666666666666, 244.44444444444446, 242.77777777777777, 243.66666666666663, 243.2222222222222, 242.66666666666666, 242.1111111111111, 243.55555555555554, 242.44444444444446, 241.44444444444443, 241.88888888888886, 242.55555555555554, 241.33333333333334, 241.77777777777777, 243.0, 242.99999999999997, 243.88888888888889, 243.77777777777774, 243.33333333333334, 243.2222222222222, 242.77777777777777, 241.55555555555557, 241.11111111111111, 361.8333333333333, 239.1111111111111, 238.55555555555554, 239.33333333333331, 239.44444444444443, 239.2222222222222, 238.33333333333334, 239.22222222222223, 239.33333333333331, 238.88888888888889, 238.66666666666666, 238.1111111111111, 238.33333333333331, 237.33333333333331, 237.41666666666666, 237.33333333333334, 237.75, 239.55555555555557, 238.55555555555554, 237.66666666666666, 236.88888888888889, 236.44444444444443, 236.11111111111111, 236.1111111111111, 237.0, 236.44444444444443, 236.33333333333334, 237.33333333333334, 236.77777777777777, 235.88888888888889, 235.77777777777777, 235.83333333333334, 235.88888888888889, 236.22222222222223, 236.0, 236.0, 236.66666666666666, 233.88888888888886, 235.66666666666663, 236.33333333333331, 235.55555555555554, 233.99999999999997, 235.55555555555554, 235.11111111111111, 235.2222222222222, 234.66666666666666, 351.66666666666663, 236.33333333333334, 235.66666666666666, 234.77777777777774, 234.55555555555557, 234.33333333333331, 233.49999999999997, 234.55555555555554, 233.33333333333334, 234.22222222222223, 234.1111111111111, 233.66666666666663, 233.2222222222222, 233.99999999999997, 234.66666666666666, 234.33333333333334, 233.33333333333331, 233.58333333333331, 232.66666666666666, 233.88888888888889, 233.0, 233.55555555555554, 233.55555555555554, 232.33333333333334, 233.11111111111111, 232.66666666666666, 233.2222222222222, 233.44444444444443, 233.1111111111111, 233.16666666666669, 233.49999999999997, 232.77777777777774, 232.0, 233.0, 233.33333333333331, 233.88888888888889, 233.0, 234.44444444444446, 233.55555555555554, 232.88888888888889, 233.66666666666666, 233.11111111111111, 232.44444444444443, 233.11111111111111, 232.88888888888889, 351.16666666666663, 233.66666666666666, 232.44444444444443, 232.66666666666666, 310.77777777777777, 234.66666666666666, 232.88888888888889, 232.66666666666666, 233.25, 233.1111111111111, 233.5, 233.66666666666666, 233.88888888888889, 233.41666666666666, 232.44444444444443, 233.11111111111111, 233.66666666666666, 351.5, 233.44444444444443, 233.41666666666666, 233.44444444444443, 232.88888888888889, 233.66666666666666, 233.55555555555557, 351.5, 232.77777777777777, 233.88888888888889, 232.91666666666666, 233.44444444444446, 233.1111111111111, 237.77777777777777, 233.55555555555557, 233.0, 232.88888888888886, 231.44444444444443, 233.11111111111111, 233.11111111111111, 233.91666666666666, 233.44444444444443, 232.88888888888889] ("Array"), y=250) -> (x/y=w1:dbl[])
  n18 = for {
    tunnel: w16 -> [w79] mode=indexing
    tunnel: w15 -> [w78]
    tunnel: w14 -> [w80]
    tunnel: w13 -> [w46]
    tunnel: w12 -> [w75]
    tunnel: w3 -> [w59]
    tunnel: bool[] [TRUE, TRUE, TRUE, TRUE, TRUE, TRUE, TRUE, TRUE, TRUE, TRUE, TRUE, TRUE, TRUE, TRUE, TRUE, TRUE, TRUE, TRUE, TRUE, TRUE, TRUE, TRUE, TRUE, TRUE, TRUE, TRUE, TRUE, TRUE, TRUE, TRUE, TRUE, TRUE, TRUE, TRUE, TRUE, TRUE, TRUE, TRUE, TRUE, TRUE, TRUE, TRUE, TRUE, TRUE, TRUE, TRUE, TRUE, TRUE, TRUE, TRUE, TRUE, TRUE, TRUE, TRUE, TRUE, TRUE, TRUE, TRUE, TRUE, TRUE, TRUE, TRUE, TRUE, TRUE, TRUE, TRUE, TRUE, TRUE, TRUE, TRUE, TRUE, TRUE, TRUE, TRUE, TRUE, TRUE, TRUE, TRUE, TRUE, TRUE, TRUE, TRUE, TRUE, TRUE, TRUE, TRUE, TRUE, TRUE, TRUE, TRUE, TRUE, TRUE, TRUE, TRUE, TRUE, TRUE, TRUE, TRUE, TRUE, TRUE, TRUE, TRUE, TRUE, TRUE, TRUE, TRUE, TRUE, TRUE, TRUE, TRUE, TRUE, TRUE, TRUE, TRUE, TRUE, TRUE, TRUE, TRUE, TRUE, TRUE, TRUE, TRUE, TRUE, TRUE, TRUE, TRUE, TRUE, TRUE, TRUE, TRUE, TRUE, TRUE, TRUE, TRUE, TRUE, TRUE, TRUE, TRUE, TRUE, TRUE, TRUE, TRUE, TRUE, TRUE, TRUE, TRUE, TRUE, TRUE, TRUE, TRUE, TRUE, TRUE, TRUE, TRUE, TRUE, TRUE, TRUE, TRUE, TRUE, TRUE, TRUE, TRUE, TRUE, TRUE, TRUE, TRUE, TRUE, TRUE, TRUE, TRUE, TRUE, TRUE, TRUE, TRUE, TRUE, TRUE, TRUE, TRUE, TRUE, TRUE, TRUE, TRUE, TRUE, TRUE, TRUE, TRUE, TRUE, TRUE, TRUE, TRUE, TRUE, TRUE, TRUE, TRUE, TRUE, TRUE, TRUE, TRUE, TRUE, TRUE, TRUE, TRUE, TRUE, TRUE, TRUE, TRUE, TRUE, TRUE, TRUE, TRUE, TRUE, TRUE, TRUE, TRUE, TRUE, TRUE, TRUE, TRUE, TRUE, TRUE, TRUE, TRUE, TRUE, TRUE, TRUE, TRUE, TRUE, TRUE, TRUE, TRUE, TRUE, TRUE, TRUE, TRUE, TRUE, TRUE, TRUE, TRUE, TRUE, TRUE, TRUE, TRUE, TRUE, TRUE, TRUE, TRUE, TRUE, TRUE, TRUE, TRUE, TRUE, TRUE, TRUE, TRUE, TRUE, TRUE, TRUE, TRUE, TRUE, TRUE, TRUE, TRUE, TRUE, TRUE, TRUE, TRUE, TRUE, TRUE, TRUE, TRUE, TRUE, TRUE, TRUE, TRUE, TRUE, TRUE, TRUE, TRUE, TRUE, TRUE, TRUE, TRUE, TRUE, TRUE, TRUE, TRUE, TRUE, TRUE, TRUE, TRUE, TRUE, TRUE, TRUE, TRUE, TRUE, TRUE, TRUE, TRUE, TRUE, TRUE, TRUE, TRUE, TRUE, TRUE, TRUE, TRUE, TRUE, TRUE, TRUE, TRUE, TRUE, TRUE, TRUE, TRUE, TRUE, TRUE, TRUE, TRUE, TRUE, TRUE, TRUE, TRUE, TRUE, TRUE, TRUE, TRUE, TRUE, TRUE, TRUE, TRUE, TRUE, TRUE, TRUE, TRUE, TRUE, TRUE, TRUE, TRUE, TRUE, TRUE, TRUE, TRUE, TRUE, TRUE, TRUE, TRUE, TRUE, TRUE, TRUE, TRUE, TRUE, TRUE, TRUE, TRUE, TRUE, TRUE, TRUE, TRUE, TRUE, TRUE, TRUE, TRUE, TRUE, TRUE, TRUE, TRUE, TRUE, TRUE, TRUE, TRUE, TRUE, TRUE, TRUE, TRUE, TRUE, TRUE, TRUE, TRUE, TRUE, TRUE, TRUE, TRUE, TRUE, TRUE, TRUE, TRUE, TRUE, TRUE, TRUE, TRUE, TRUE, TRUE, TRUE, TRUE, TRUE, TRUE, TRUE, TRUE, TRUE, TRUE, TRUE, TRUE, TRUE, TRUE, TRUE, TRUE, TRUE, TRUE, TRUE, TRUE, TRUE, TRUE, TRUE, TRUE, TRUE, TRUE, TRUE, TRUE, TRUE, TRUE, TRUE, TRUE, TRUE, TRUE, TRUE, TRUE, TRUE, TRUE, TRUE, TRUE, TRUE, TRUE, TRUE, TRUE, TRUE, TRUE, TRUE, TRUE, TRUE, TRUE, TRUE, TRUE, TRUE, TRUE, TRUE, TRUE, TRUE, TRUE, TRUE, TRUE, TRUE, TRUE, TRUE, TRUE, TRUE, TRUE, TRUE, TRUE, TRUE, TRUE, TRUE, TRUE, TRUE, TRUE, TRUE, TRUE, TRUE, TRUE, TRUE, TRUE, TRUE, TRUE, TRUE, TRUE, TRUE, TRUE, TRUE, TRUE, TRUE, TRUE, TRUE, TRUE, TRUE, TRUE, TRUE, TRUE, TRUE, TRUE, TRUE, TRUE, TRUE, TRUE, TRUE, TRUE, TRUE, TRUE, TRUE, TRUE, TRUE, TRUE, TRUE, TRUE, TRUE, TRUE, TRUE, TRUE, TRUE, TRUE, TRUE, TRUE, TRUE, TRUE, TRUE, TRUE, TRUE, TRUE, TRUE, TRUE, TRUE, TRUE, TRUE, TRUE, TRUE, TRUE, TRUE, TRUE, TRUE, TRUE, TRUE, TRUE, TRUE, TRUE, TRUE, TRUE, TRUE, TRUE, TRUE, TRUE, TRUE, TRUE, TRUE, TRUE, TRUE, TRUE, TRUE, TRUE, TRUE, TRUE, TRUE, TRUE, TRUE, TRUE, TRUE, TRUE, TRUE, TRUE, TRUE, TRUE, TRUE, TRUE, TRUE, TRUE, TRUE, TRUE, TRUE, TRUE, TRUE, TRUE, TRUE, TRUE, TRUE, TRUE, TRUE, TRUE, TRUE, TRUE, TRUE, TRUE, TRUE, TRUE, TRUE, TRUE, TRUE, TRUE, TRUE, TRUE, TRUE, TRUE, TRUE, TRUE, TRUE, TRUE, TRUE, TRUE, TRUE, TRUE, TRUE, TRUE, TRUE, TRUE, TRUE, TRUE, TRUE, TRUE, TRUE, TRUE, TRUE, TRUE, TRUE, TRUE, TRUE, TRUE, TRUE, TRUE, TRUE, TRUE, TRUE, TRUE, TRUE, TRUE, TRUE, TRUE, TRUE, TRUE, TRUE, TRUE, TRUE, TRUE, TRUE, TRUE, TRUE, TRUE, TRUE, TRUE, TRUE, TRUE, TRUE, TRUE, TRUE, TRUE, TRUE, TRUE, TRUE, TRUE, TRUE, TRUE, TRUE, TRUE, TRUE, TRUE, TRUE, TRUE, TRUE, TRUE, TRUE, TRUE, TRUE, TRUE, TRUE, TRUE, TRUE, TRUE, TRUE, TRUE, TRUE, TRUE, TRUE, TRUE, TRUE, TRUE, TRUE, TRUE, TRUE, TRUE, TRUE, FALSE, FALSE, FALSE, FALSE, FALSE, FALSE, FALSE, FALSE, FALSE, FALSE, FALSE, FALSE, FALSE, FALSE, FALSE, FALSE, FALSE, FALSE, FALSE, FALSE, FALSE, FALSE, FALSE, FALSE, FALSE, FALSE, FALSE, FALSE, FALSE, FALSE, FALSE, FALSE, FALSE, FALSE, FALSE, FALSE, FALSE, FALSE, FALSE, FALSE, FALSE, FALSE, FALSE, FALSE, FALSE, FALSE, FALSE, FALSE, FALSE, FALSE, TRUE, TRUE, TRUE, TRUE, TRUE, TRUE, TRUE, TRUE, TRUE, TRUE, TRUE, TRUE, TRUE, TRUE, TRUE, TRUE, TRUE, TRUE, TRUE, TRUE, TRUE, TRUE, TRUE, TRUE, TRUE, FALSE, FALSE, FALSE, FALSE, FALSE, FALSE, FALSE, FALSE, FALSE, FALSE, FALSE, FALSE, FALSE, FALSE, FALSE, FALSE, FALSE, FALSE, FALSE, FALSE, FALSE, FALSE, FALSE, FALSE, FALSE, FALSE, FALSE, FALSE, FALSE, FALSE, FALSE, FALSE, FALSE, FALSE, FALSE, FALSE, FALSE, FALSE, FALSE, FALSE, FALSE, FALSE, FALSE, FALSE, FALSE, FALSE, FALSE, FALSE, FALSE, FALSE, FALSE, FALSE, FALSE, FALSE, FALSE, FALSE, FALSE, FALSE, FALSE, FALSE, FALSE, FALSE, FALSE, FALSE, FALSE, FALSE, FALSE, FALSE, FALSE, FALSE, FALSE, FALSE, FALSE, FALSE, FALSE, FALSE, FALSE, FALSE, FALSE, FALSE, FALSE, FALSE, FALSE, FALSE, FALSE, FALSE, FALSE, FALSE, FALSE, FALSE, FALSE, FALSE, FALSE, FALSE, FALSE, FALSE, FALSE, FALSE, FALSE, FALSE, FALSE, FALSE, FALSE, FALSE, FALSE, FALSE, FALSE, FALSE, FALSE, FALSE, FALSE, FALSE, FALSE, FALSE, FALSE, FALSE, FALSE, FALSE, FALSE, FALSE, FALSE, FALSE, FALSE, FALSE, FALSE, FALSE, FALSE, FALSE, FALSE, FALSE, FALSE, FALSE, FALSE, FALSE, FALSE, FALSE, FALSE, FALSE, FALSE, FALSE, FALSE, FALSE, FALSE, FALSE, FALSE, FALSE, FALSE, FALSE, FALSE, FALSE, FALSE, FALSE, FALSE, FALSE, FALSE, FALSE, FALSE, FALSE, FALSE, FALSE, FALSE, FALSE, FALSE, FALSE, FALSE, FALSE, FALSE, FALSE, FALSE, FALSE, FALSE, FALSE, FALSE, FALSE, FALSE, FALSE, FALSE, FALSE, FALSE, FALSE, FALSE, FALSE, FALSE, FALSE, FALSE, FALSE, FALSE, FALSE, FALSE, FALSE, FALSE, FALSE, FALSE, FALSE, FALSE, FALSE, FALSE, FALSE, FALSE, FALSE, FALSE, FALSE, FALSE, FALSE, FALSE, FALSE, FALSE, FALSE, FALSE, FALSE, FALSE, FALSE, FALSE, FALSE, FALSE, FALSE, FALSE, FALSE, FALSE, FALSE, FALSE, FALSE, FALSE, FALSE, FALSE, FALSE, FALSE, FALSE, FALSE, FALSE, FALSE, FALSE, FALSE, FALSE, FALSE, FALSE, FALSE, FALSE, FALSE, FALSE, FALSE, FALSE, FALSE, FALSE, FALSE, FALSE, FALSE, FALSE, FALSE, FALSE, FALSE, FALSE, FALSE, FALSE, FALSE, FALSE, FALSE, FALSE, FALSE, FALSE, FALSE, FALSE, FALSE, FALSE, FALSE, FALSE, FALSE, FALSE, FALSE, FALSE, FALSE, FALSE, FALSE, FALSE, FALSE, FALSE, FALSE, FALSE, FALSE, FALSE, FALSE, FALSE, FALSE, FALSE, FALSE, FALSE, FALSE, FALSE, FALSE, FALSE, FALSE, FALSE, FALSE, FALSE, FALSE, FALSE, FALSE, FALSE, FALSE, FALSE, FALSE, FALSE, FALSE, FALSE, FALSE, FALSE, FALSE, FALSE, FALSE, FALSE, FALSE, FALSE, FALSE, FALSE, FALSE, FALSE, FALSE, FALSE, FALSE, FALSE, FALSE, FALSE, FALSE, FALSE, FALSE, FALSE, FALSE, FALSE, FALSE, FALSE, FALSE, FALSE, FALSE, FALSE, FALSE, FALSE, FALSE, FALSE, FALSE, FALSE, FALSE, FALSE, FALSE, FALSE, FALSE, FALSE, FALSE, FALSE, FALSE, FALSE, FALSE, FALSE, FALSE, FALSE, FALSE, FALSE, FALSE, FALSE, FALSE, FALSE, FALSE, FALSE, FALSE, FALSE, FALSE, FALSE, FALSE, FALSE, FALSE, FALSE, FALSE, FALSE, FALSE, FALSE, FALSE, FALSE, FALSE, FALSE, FALSE, FALSE, FALSE, FALSE, FALSE, FALSE, FALSE, FALSE, FALSE, FALSE, FALSE, FALSE, FALSE, FALSE, FALSE, FALSE, FALSE, FALSE, FALSE, FALSE, FALSE, FALSE, FALSE, FALSE, FALSE, FALSE, FALSE, FALSE, FALSE, FALSE, FALSE, FALSE, FALSE, FALSE, FALSE, FALSE, FALSE, FALSE, FALSE, FALSE, FALSE, FALSE, FALSE, FALSE, FALSE, FALSE, FALSE, FALSE, FALSE, FALSE, FALSE, FALSE, FALSE, FALSE, FALSE, FALSE, FALSE, FALSE, FALSE, FALSE, FALSE, FALSE, FALSE, FALSE, FALSE, FALSE, FALSE, FALSE, FALSE, FALSE, FALSE, FALSE, FALSE, FALSE, FALSE, FALSE, FALSE, FALSE, FALSE, FALSE, FALSE, FALSE, FALSE, FALSE, FALSE, FALSE, FALSE, FALSE, FALSE, FALSE, FALSE, FALSE, FALSE, FALSE, FALSE, FALSE, FALSE, FALSE, FALSE, FALSE, FALSE, FALSE, FALSE, FALSE, FALSE, FALSE, FALSE, FALSE, FALSE, FALSE, FALSE, FALSE, FALSE, FALSE, FALSE, FALSE, FALSE, FALSE, FALSE, FALSE, FALSE, FALSE, FALSE, FALSE, FALSE, FALSE, FALSE, FALSE, FALSE, FALSE, FALSE, FALSE, FALSE, FALSE, FALSE, FALSE, FALSE, FALSE, FALSE, FALSE, FALSE, FALSE, FALSE, FALSE, FALSE, FALSE, FALSE, FALSE, FALSE, FALSE, FALSE, FALSE, FALSE, FALSE, FALSE, FALSE, FALSE, FALSE, FALSE, FALSE, FALSE, FALSE, FALSE, FALSE, FALSE, FALSE, FALSE, FALSE, FALSE, FALSE, FALSE, FALSE, FALSE, FALSE, FALSE, FALSE, FALSE, FALSE, FALSE, FALSE, FALSE, FALSE, FALSE, FALSE, FALSE, FALSE, FALSE, FALSE, FALSE, FALSE, FALSE, FALSE, FALSE, FALSE, FALSE, FALSE, FALSE, FALSE, FALSE, FALSE, FALSE, FALSE, FALSE, FALSE, FALSE, FALSE, FALSE, FALSE, FALSE, FALSE, FALSE, FALSE, FALSE, FALSE, FALSE, FALSE, FALSE, FALSE, FALSE, FALSE, FALSE, FALSE, FALSE, FALSE, FALSE, FALSE, FALSE, FALSE, FALSE, FALSE, FALSE, FALSE, FALSE, FALSE, FALSE, FALSE, FALSE, FALSE, FALSE, FALSE, FALSE, FALSE, FALSE, FALSE, FALSE, FALSE, FALSE, FALSE, FALSE, FALSE, FALSE, FALSE, FALSE, FALSE, FALSE, FALSE, FALSE, FALSE, FALSE, FALSE, FALSE, FALSE, FALSE, FALSE, FALSE, FALSE, FALSE, FALSE, FALSE, FALSE, FALSE, FALSE, FALSE, FALSE, FALSE, FALSE, FALSE, FALSE, FALSE, FALSE, FALSE, FALSE, FALSE, FALSE, FALSE, FALSE, FALSE, FALSE, FALSE, FALSE, FALSE, FALSE, FALSE, FALSE, FALSE, FALSE, FALSE, FALSE, FALSE, FALSE, FALSE, FALSE, FALSE, FALSE, FALSE, FALSE, FALSE, FALSE, FALSE, FALSE, FALSE, FALSE, FALSE, FALSE, FALSE, FALSE, FALSE, FALSE, FALSE, FALSE, FALSE, FALSE, FALSE, FALSE, FALSE, FALSE, FALSE, FALSE, FALSE, FALSE, FALSE, FALSE, FALSE, FALSE, FALSE, FALSE, FALSE, FALSE, FALSE, FALSE, FALSE, FALSE, FALSE, FALSE, FALSE, FALSE, FALSE, FALSE, FALSE, FALSE, FALSE, FALSE, FALSE, FALSE, FALSE, FALSE, FALSE, FALSE, FALSE, FALSE, FALSE, FALSE, FALSE, FALSE, FALSE, FALSE, FALSE, FALSE, FALSE, FALSE, FALSE, FALSE, TRUE] ("Resp Gate") -> [w37]
    tunnel: w8 -> [w39]
    tunnel: bool[][] array161x1000[161000 elements] ("Resp Gate") -> [w38]
    tunnel: w1 -> [w36]
    n19 = Index Array(array=w78, index=w79) -> (element=w77:string)
    n20 = Match Pattern(string=w77, regular expression=w80) -> (before substring=w62:string, after substring=w61:string)  [unwired: 3 out]
    n21 = Initialize Array(FALSE, 80 ("dimension size")) -> (w35:bool[])
    n22 = Concatenate Strings(w62, "*" ("prompt"), w61) -> (w60:string)
    "Root Name" <- w60
    n23 = List Folder(path=w46, pattern=w60) -> (filenames=w45:string[])  [unwired: 1 in, 4 out]
    n24 = Index Array(array=w45) -> (element=w44:string)  [unwired: 1 in]
    n25 = Build Path(base path=w46, name or relative path=w44) -> (appended path=w43:path)
    n26 = call "ReadHeadFast.vi"("new file path"=w43) -> ("A/D info"=w42:T3)  [unwired: 2 in, 16 out]
    n27 = Concatenate Strings("RET" ("prompt"), w62) -> (w73:string)
    n28 = Unbundle By Name(w42) -> ("# lines per scan"=w41:u16)
    n29 = Index Array(array=w45) -> (element=w72:string)  [unwired: 1 in]
    n30 = Array Size(array=w45) -> (size(s)=w64:i32)
    n31 = Build Path(base path=w46, name or relative path=w72) -> (appended path=w71:path)
    n32 = call "ReadHead.vi"("new file path"=w71) -> ("Header In"=w65:T4, "Pan Scan Settings"=w68:T5)  [unwired: 17 out]
    n33 = Unbundle By Name(w65) -> ("header info.Head length"=w51:i16, "A/D info.# rf points per line"=w57:u16, "A/D info.# A/D bits"=w50:i16)
    n34 = Unbundle By Name(w68) -> ("Distance between\nscan planes (mm)"=w67:u16)
    n35 = Bundle By Name(cluster=w65, "A/D info.# lines per scan"=w64, "Scan Settings.Distance between\nscan planes (um)"=u16 0 ("Scan Settings.Distance between\nscan planes (mm)"), "Scan Settings.Distance between\nscan lines (um)"=w67) -> (w70:T4)
    n36 = Greater?(x=w50, y=u16 8) -> (0:w55:bool)
    n37 = Select(t=u16 2 ("y"), s=w55, f=u16 1 ("y")) -> (s? t:f=w54:u16)
    n38 = Compound Arithmetic op=MULTIPLY(w54, w57) -> (w58:u16)
    n39 = Compound Arithmetic op=MULTIPLY(w58, w64) -> (w49:i32)
    n40 = Add(x=w51, y=w49) -> (x+y=w63:i32)
    n41 = call "MakeHeader.vi"("Header In"=w70) -> ("Header String"=w69:string)  [unwired: 6 out]
    n42 = stacked-sequence {
      seq-local: [w87 _ _] -> [_ w134 w221]
      tunnel: w75 -> [w91 _ _]
      tunnel: w73 -> [w90 _ _]
      tunnel: w46 -> [_ w139 _]
      tunnel: w45 -> [_ w138 _]
      tunnel: w69 -> [w89 _ _]
      tunnel: w63 -> [w84 _ _]
      tunnel: w61 -> [w88 _ _]
      tunnel: w59 -> [_ w137 _]
      tunnel: w58 -> [_ w136 _]
      tunnel: w51 -> [_ w135 _]
      tunnel: w41 -> [w81 w132 _]
      tunnel: w50 -> [w86 w133 _]
      tunnel: w49 -> [w82 _ _]
      tunnel: w38 -> [_ w127 _]
      tunnel: 600 -> [_ w131 _]
      tunnel: w39 -> [_ w130 _]
      tunnel: w37 -> [_ w129 _]
      tunnel: w36 -> [_ w128 _]
      tunnel: w35 -> [_ w126 _]
      frame #0 {
        n43 = Initialize Array(i16 0, w82) -> (w83:i16[])
        n44 = for {
          N: w81 -> [_]
          tunnel: w91 -> [w113]
          tunnel: w90 -> [w109]
          tunnel: w89 -> [w107]
          tunnel: w84 -> [w106]
          tunnel: w88 -> [w105]
          tunnel: [w92] -> w87 mode=indexing
          tunnel: w86 -> [w96]
          tunnel: w83 -> [w95]
          i -> [w97]
          n45 = call "NumberFileName.vi"("String"=w105, "File number"=w97, "file name"=w109) -> ("Numbered File"=w108:string)  [unwired: 1 in]
          n46 = Build Path(base path=w113, name or relative path=w108) -> (appended path=w112:path)
          n47 = Open/Create/Replace File(file path (use dialog)=w112, operation (0:open)=T1."replace or create") -> (refnum out=w110:refnum<file>, error out=w104:errorcluster)  [unwired: 1 in, 4 out]
          n48 = Set File Size(4:w104, 6:w106, 7:w110) -> (0:w101:errorcluster, 3:w102:refnum<file>)
          n49 = Set File Position(refnum=w102, from (0:start)=enum16{"start", "end", "current"}."start", error in=w101) -> (refnum out=w100:refnum<file>, error out=w99:errorcluster)  [unwired: 1 in]
          n50 = Write to Binary File(file (use dialog)=w100, data=w107, error in=w99, 5:FALSE ("prepend array or string size? (T)")) -> (refnum out=w93:refnum<file>, error out=w94:errorcluster)  [unwired: 3 out]
          n51 = case shown="0, Default" w96 {
            tunnel: w93 -> [w119 w124]
            tunnel: w94 -> [w118 w123]
            tunnel: w95 -> [w115 w120]
            tunnel: [w114 w121] -> w92
            frame 0, Default {
              n52 = Write to Binary File(file (use dialog)=w119, data=w115, error in=w118, 5:FALSE ("prepend array or string size? (T)"), 9:T2."little-endian" ("byte order (0:big-endian, network order)")) -> (refnum out=w114:refnum<file>)  [unwired: 3 out]
            }
            frame 8 {
              n53 = To Byte Integer(number=w120) -> (8bit integer=w122:i8[])
              n54 = Write to Binary File(file (use dialog)=w124, data=w122, error in=w123, 5:FALSE ("prepend array or string size? (T)")) -> (refnum out=w121:refnum<file>)  [unwired: 1 in, 3 out]
            }
          }
        }
      }
      frame #1 {
        n55 = for {
          tunnel: w139 -> [w159]
          tunnel: w138 -> [w158] mode=indexing
          tunnel: w136 -> [w157]
          tunnel: w137 -> [w145] mode=indexing
          tunnel: w135 -> [w156]
          tunnel: w134 -> [w154]
          tunnel: w133 -> [w152]
          tunnel: w132 -> [w148]
          tunnel: w131 -> [w147]
          tunnel: w130 -> [w146] mode=indexing
          tunnel: w129 -> [w142]
          tunnel: w128 -> [w143] mode=indexing
          tunnel: w127 -> [w140] mode=indexing
          tunnel: w126 -> [w141]
          i -> [w153]
          # "Read from M mode"
          n56 = Build Path(base path=w159, name or relative path=w158) -> (appended path=w155:path)
          n57 = Replace Array Subset(array=w140, new element=w141) -> ()  [unwired: 1 in, 1 out]
          n58 = Build Array (concatenate)(w146, w145) -> ()  [unwired: 1 out]
          n59 = call "ReadEyeFile.vi"("new file path"=w155) -> ("2-D data array"=w150:i16[][], "# lines per scan"=w149:u16)  [unwired: 1 in, 16 out]
          "Raw data" <- w150
          n60 = Reverse 1D Array(array=w145) -> (reversed array=w144:dbl[])
          n61 = Or(x=w142, y=FALSE) -> ()  [unwired: 1 out]
          n62 = for {
            tunnel: w157 -> [w168]
            tunnel: w144 -> [w166] mode=indexing
            tunnel: w150 -> [w170]
            tunnel: w140 -> [w169]
            tunnel: w156 -> [w167]
            tunnel: w154 -> [w165]
            tunnel: w153 -> [w164]
            tunnel: w152 -> [w163]
            tunnel: w149 -> [w162]
            tunnel: w148 -> [w161]
            tunnel: w147 -> [_]
            tunnel: w143 -> [w160]
            # "Move through each heart beat"
            n63 = case shown="10, Default" w166 {
              tunnel: w170 -> [_ w181]
              tunnel: w169 -> [_ w180]
              tunnel: w168 -> [_ w179]
              tunnel: w167 -> [_ w178]
              tunnel: w166 -> [_ w177]
              tunnel: w165 -> [_ w176]
              tunnel: w164 -> [_ w175]
              tunnel: w163 -> [_ w174]
              tunnel: w162 -> [_ w173]
              tunnel: w161 -> [_ w172]
              tunnel: w160 -> [_ w171]
              frame 0..3 {
                # "If no EKG index. Skip"
              }
              frame 10, Default {
                n64 = for {
                  N: w172 -> [_]
                  tunnel: w181 -> [w203]
                  tunnel: w177 -> [w197]
                  tunnel: w180 -> [w198]
                  tunnel: w179 -> [w202]
                  tunnel: w178 -> [w200]
                  tunnel: w176 -> [w196] mode=indexing
                  tunnel: w175 -> [w194]
                  tunnel: w174 -> [w191]
                  tunnel: w173 -> [w187]
                  tunnel: w171 -> [w183]
                  i -> [w184]
                  # "Insert into B-mode"
                  n65 = Decrement(x=w187) -> (x-1=w190:u16)
                  n66 = Multiply(x=w184, y=w183) -> (x*y=w182:dbl)
                  n67 = Add(x=w182, y=w197) -> (x+y=w193:dbl)
                  n68 = In Range and Coerce(upper limit=w190, x=w193, lower limit=0.0 ("upper limit")) -> (coerced(x)=w188:dbl, In Range?=w186:bool)
                  n69 = Multiply(x=w194, y=w202) -> (x*y=w201:i32)
                  n70 = Add(x=w201, y=w200) -> (x+y=w199:i32)
                  n71 = Index Array(array=w198, index=w188) -> (element=w195:bool)
                  n72 = And(x=w186, y=w195) -> (x .and. y?=w185:bool)
                  n73 = Index Array(array=w203, index (row)=w188) -> (element=w189:i16[])  [unwired: 1 in]
                  n74 = case shown="True" w185 {
                    tunnel: w199 -> [_ w210]
                    tunnel: w196 -> [_ w209]
                    tunnel: w191 -> [_ w208]
                    tunnel: w189 -> [_ w204]
                    frame False {
                    }
                    frame True {
                      n75 = Set File Position(offset (in bytes) (0)=w210, refnum=w209, from (0:start)=enum16{"start", "end", "current"}."start") -> (refnum out=w206:refnum<file>, error out=w205:errorcluster)  [unwired: 1 in]
                      n76 = case shown="0, Default" w208 {
                        tunnel: w204 -> [w215 w219]
                        tunnel: w206 -> [w214 w218]
                        tunnel: w205 -> [w213 w217]
                        frame 0, Default {
                          n77 = Write to Binary File(file (use dialog)=w214, data=w215, error in=w213, 5:FALSE ("prepend array or string size? (T)"), 9:T2."little-endian" ("byte order (0:big-endian, network order)")) -> ()  [unwired: 4 out]
                        }
                        frame 8 {
                          n78 = To Byte Integer(number=w219) -> (8bit integer=w216:i8[])
                          n79 = Write to Binary File(file (use dialog)=w218, data=w216, error in=w217, 5:FALSE ("prepend array or string size? (T)")) -> ()  [unwired: 1 in, 4 out]
                        }
                      }
                    }
                  }
                }
              }
            }
          }
          "File num" <- w153
        }
      }
      frame #2 {
        n80 = for {
          tunnel: w221 -> [w222] mode=indexing
          n81 = Close File(refnum=w222) -> ()  [unwired: 1 in, 2 out]
        }
      }
    }
  }
